vi "1D Scan.vi"(7 "Dwell Time (ms)":i32=10, 8 "Num Steps":i32, 9 "Step":dbl, 10 "Min":dbl, 11 "Channel":tag) -> (3 "Counts":i32[](array[numeric]))   [LabVIEW 2012]
uses:
  <vilib>/DAQmx/write.llb/DAQmx Write (Analog DBL 1Chan 1Samp).vi
  <vilib>/DAQmx/read.llb/DAQmx Read (Counter U32 1Chan 1Samp).vi
  <vilib>/DAQmx/create/channels.llb/DAQmx Create Channel (AO-Voltage-Basic).vi
  Channels.vi
  <vilib>/DAQmx/create/channels.llb/DAQmx Create Channel (CI-Count Edges).vi
  <vilib>/DAQmx/miscellaneous.llb/DAQmx Fill In Error Info.vi
  Global Vars.vi
panel:
  out "AO Voltage":dbl
  in  "Abort":bool
  out "Total Count":u32
  out "Current Count":i32
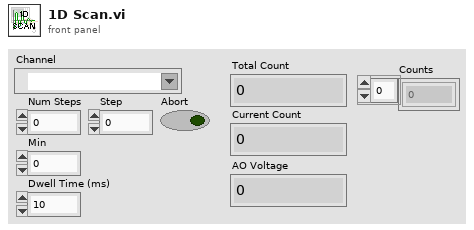
[diagram p1: front panel]
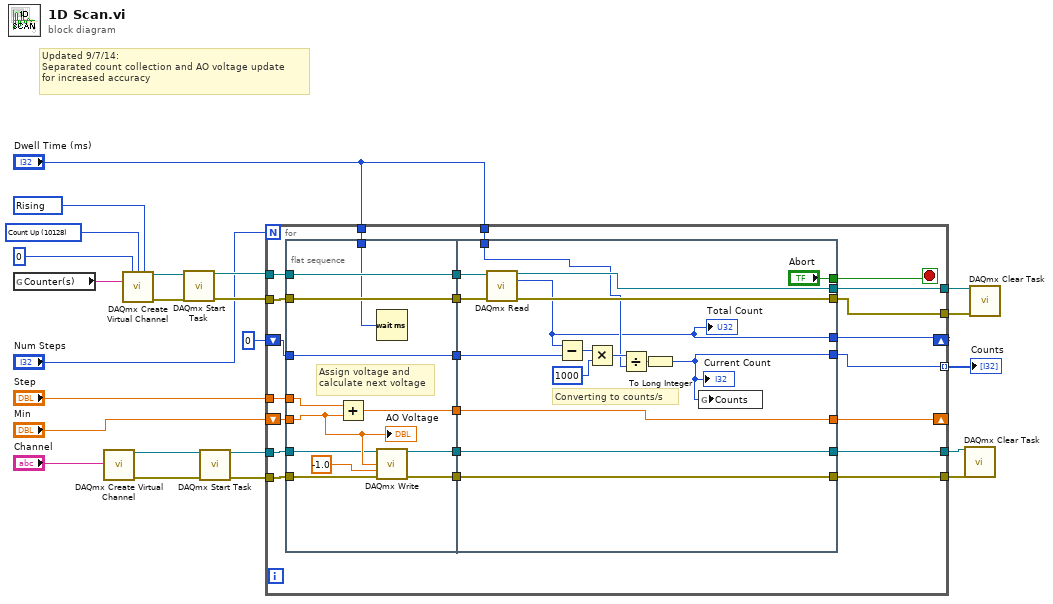
[diagram p0: block diagram]
diagram:
  w16 = 10280 items=["Rising"=10280, "Falling"=10171] ("Edge")
  w17 = 10128 items=["Count Up"=10128, "Count Down"=10124, "Externally Controlled"=10326] ("Count Direction")
  # "Updated 9/7/14:\nSeparated count collection and AO voltage update\nfor increased accuracy"
  n1 = global read "Channels.vi" "Counter(s)"() -> (w15:tag)
  n2 = call-poly <vilib>:"DAQmx Create Virtual Channel.vi"("physical channels"="Channel") -> ("task out"=w22:refnum<k21>, "error out"=w21:errorcluster)  [unwired: 13 in]
  n3 = call-poly <vilib>:"DAQmx Create Virtual Channel.vi"("initial count"=u32 0 ("Initial Count"), "count direction"=w17, "edge"=w16, "counter"=w15) -> ("task out"=w14:refnum<k21>, "error out"=w12:errorcluster)  [unwired: 10 in]
  n4 = call <vilib>:"DAQmx Start Task.vi"("task/channels in"=w14, "error in"=w12) -> ("task out"=w13:refnum<k21>, "error out"=w11:errorcluster)  [unwired: 12 in]
  n5 = call <vilib>:"DAQmx Start Task.vi"("task/channels in"=w22, "error in"=w21) -> ("task out"=w20:refnum<k21>, "error out"=w19:errorcluster)  [unwired: 12 in]
  n6 = for {
    N: "Num Steps" -> [_]
    shift-right: [w28] -> _
    shift-left: "Min" -> [w44]
    shift-right: [w36] -> _
    shift-left: 0 -> [w40]
    tunnel: w20 -> [w46]
    tunnel: w19 -> [w45]
    tunnel: w13 -> [w42]
    tunnel: w11 -> [w41]
    tunnel: "Step" -> [w43]
    tunnel: "Dwell Time (ms)" -> [w37]
    tunnel: [w39] -> w7
    tunnel: [w38] -> w6
    tunnel: [w35] -> w4 mode=indexing
    tunnel: [w27] -> w3
    tunnel: [w26] -> w2
    tunnel: "Dwell Time (ms)" -> [w25]
    stop <- w24 stop-if-true
    n7 = flat-sequence {
      tunnel: w44 -> [w53]
      tunnel: w43 -> [w54]
      tunnel: w40 -> [w56]
      tunnel: w41 -> [w57]
      tunnel: w42 -> [w58]
      tunnel: w45 -> [w48]
      tunnel: w46 -> [w49]
      tunnel: [w51] -> w34
      tunnel: [w50] -> w33
      tunnel: [w58] -> w32
      tunnel: [w57] -> w31
      tunnel: [w56] -> w30
      tunnel: [w52] -> w29
      tunnel: w25 -> [w47]
      tunnel: w37 -> [w63]
      tunnel: w34 -> [w74]
      tunnel: w33 -> [w73]
      tunnel: w32 -> [w68]
      tunnel: w31 -> [w67]
      tunnel: w30 -> [w66]
      tunnel: w29 -> [w60]
      tunnel: [w74] -> w27
      tunnel: [w73] -> w26
      tunnel: [w65] -> w39
      tunnel: [w64] -> w38
      tunnel: [w62] -> w36
      tunnel: [w61] -> w35
      tunnel: [w60] -> w28
      tunnel: ["Abort"] -> w24
      frame #0 {
        # "Assign voltage and\ncalculate next voltage"
        n8 = Add(x=w54, y=w53) -> (x+y=w52:dbl)
        n9 = Wait (ms)(milliseconds to wait=w47) -> ()  [unwired: 1 out]
        n10 = call-poly <vilib>:"DAQmx Write.vi"("task/channels in"=w49, "data"=w53, "timeout"=-1.0, "error in"=w48) -> ("task out"=w51:refnum<k21>, "error out"=w50:errorcluster)  [unwired: 9 in, 1 out]
        "AO Voltage" <- w53
      }
      frame #1 {
        # "Converting to counts/s"
        n11 = call-poly <vilib>:"DAQmx Read.vi"("task/channels in"=w68, "error in"=w67) -> ("task out"=w65:refnum<k21>, "data"=w62:u32, "error out"=w64:errorcluster)  [unwired: 11 in]
        "Total Count" <- w62
        n12 = Subtract(x=w62, y=w66) -> (x-y=w69:u32)
        n13 = Multiply(x=w69, y=1000) -> (x*y=w71:u32)
        n14 = Divide(x=w71, y=w63) -> (x/y=w72:dbl)
        n15 = To Long Integer(number=w72) -> (32bit integer=w61:i32)
        "Current Count" <- w61
        n16 = global write "Global Vars.vi" "Counts"(w61) -> ()
      }
    }
  }
  "Counts" <- w4
  n17 = call <vilib>:"DAQmx Clear Task.vi"("task in"=w3, "error in"=w2) -> ()  [unwired: 13 in, 1 out]
  n18 = call <vilib>:"DAQmx Clear Task.vi"("task in"=w7, "error in"=w6) -> ()  [unwired: 13 in, 1 out]
